vi "Is Reference Changed.vi"(8 "error in (no error)":errorcluster, 11 "Generator in":refnum<class "Generator.lvclass">) -> (0 "error out":errorcluster, 2 "REF frequency or phase changed?":bool, 3 "Generator out":refnum<class "Generator.lvclass">)   [LabVIEW 2019, in "Generator.lvclass"]
uses:
  Generator.lvclass
  Generator.lvclass/Generator.ctl
  0a297234-f1a7-4d57-8c2f-a53db9f138df.vi
  5b7423eb-c88a-4eec-af7d-cb9347c02f62.vi
  12c8d0f8-d186-41bb-9798-d6bc036f444e.vi
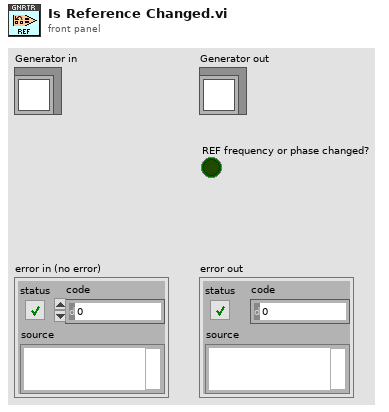
[diagram p1: front panel]
types:
  T1 = cluster{"Enable?":bool, "Channel":i32, "Frequency":dbl, "Phase":dbl, "TC":dbl, "Roll-Off":i32}[]
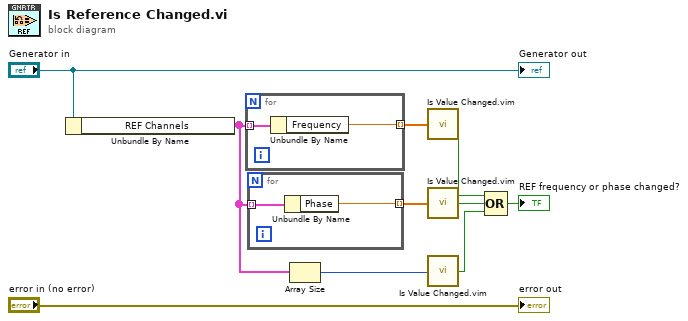
[diagram p0: block diagram]
diagram:
  n1 = Unbundle By Name("Generator in") -> ("REF Channels"=w7:T1)
  n2 = for {
    tunnel: w7 -> [w12] mode=indexing
    tunnel: [w11] -> w3 mode=indexing
    n3 = Unbundle By Name(w12) -> ("Frequency"=w11:dbl)
  }
  n4 = for {
    tunnel: w7 -> [w14] mode=indexing
    tunnel: [w13] -> w4 mode=indexing
    n5 = Unbundle By Name(w14) -> ("Phase"=w13:dbl)
  }
  n6 = Array Size(array=w7) -> (size(s)=w6:i32)
  n7 = call "Is Value Changed.vim"("value"=w3) -> ("changed or first call?"=w2:bool)
  n8 = call "Is Value Changed.vim"("value"=w4) -> ("changed or first call?"=w1:bool)
  n9 = call "Is Value Changed.vim"("value"=w6) -> ("changed or first call?"=w5:bool)
  n10 = Compound Arithmetic op=OR(w2, w1, w5) -> (→"REF frequency or phase changed?":bool)
  "error out" <- "error in (no error)"
  "Generator out" <- "Generator in"
